vi "Message Check.vi"(8 "error in (no error)":errorcluster, 10 "element":cluster{"ID":string, "current time":timestamp}[](array[cluster]), 11 "Array in":refnum<class "Button.lvclass">[](array[class])) -> (0 "error out":errorcluster, 3 "Array":refnum<class "Button.lvclass">[](array[class]))   [LabVIEW 2018]
uses:
  Button Class/Button.lvclass
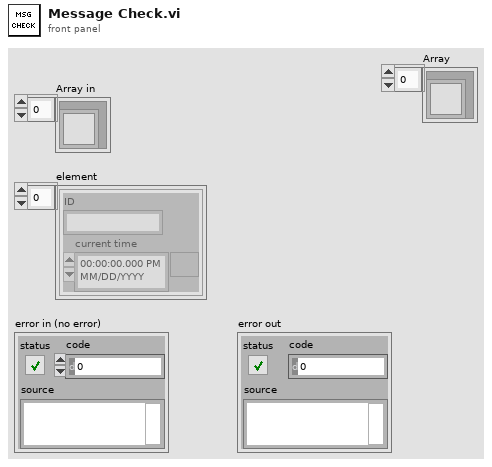
[diagram p1: front panel]
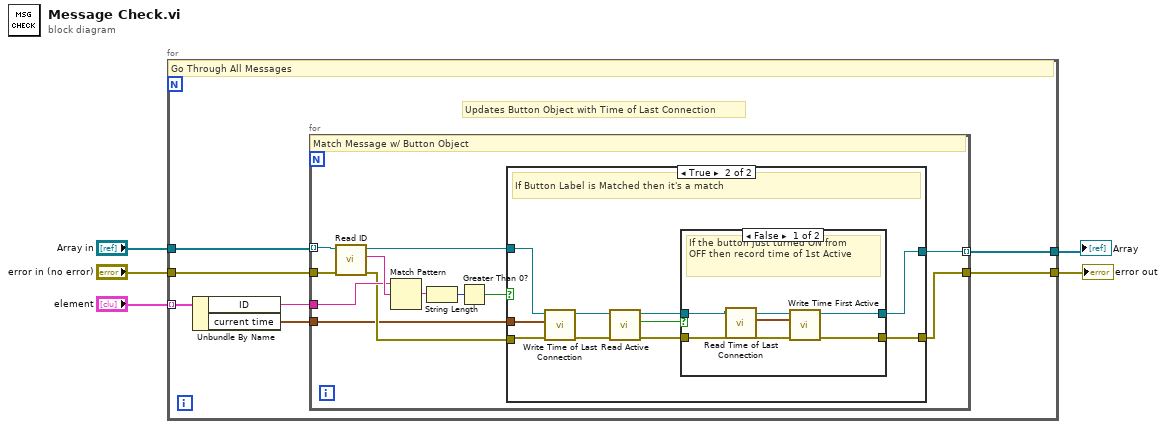
[diagram p0: block diagram]
diagram:
  n1 = for {
    tunnel: "element" -> [w12] mode=indexing
    tunnel: "Array in" -> [w11]
    tunnel: [w8] -> w5
    tunnel: "error in (no error)" -> [w7]
    tunnel: [w6] -> w1
    # "Updates Button Object with Time of Last Connection"
    # "Go Through All Messages"
    n2 = Unbundle By Name(w12) -> ("ID"=w10:string, "current time"=w9:timestamp)
    n3 = for {
      tunnel: w11 -> [w24] mode=indexing
      tunnel: w10 -> [w21]
      tunnel: w9 -> [w16]
      tunnel: [w15] -> w8
      tunnel: w7 -> [w23]
      tunnel: [w13] -> w6 mode=indexing
      # "Match Message w/ Button Object"
      n4 = call-dynamic "Read ID.vi"("error in (no error)"=w23, "Button in"=w24) -> ("error out"=w17:errorcluster, "ID"=w22:string, "Button out"=w18:refnum<class "Button.lvclass">)  [unwired: 7 in]
      n5 = Match Pattern(string=w21, regular expression=w22) -> (match substring=w19:string)  [unwired: 1 in, 3 out]
      n6 = String Length(string=w19) -> (length=w20:i32)
      n7 = Greater Than 0?(x=w20) -> (x > 0?=w14:bool)
      n8 = case shown="True" w14 {
        tunnel: w18 -> [w25 w36]
        tunnel: w17 -> [w26 w35]
        tunnel: w16 -> [_ w34]
        tunnel: [w26 w28] -> w15
        tunnel: [w25 w27] -> w13
        frame False {
          # "Not a Match"
        }
        frame True {
          # "If Button Label is Matched then it's a match"
          n9 = call-dynamic "Write Time of Last Connection.vi"("error in (no error)"=w35, "Time of Last Connection"=w34, "Button in"=w36) -> ("error out"=w33:errorcluster, "Button out"=w32:refnum<class "Button.lvclass">)  [unwired: 7 in]
          n10 = call-dynamic "Read Active.vi"("error in (no error)"=w33, "Button in"=w32) -> ("error out"=w29:errorcluster, "Active"=w31:bool, "Button out"=w30:refnum<class "Button.lvclass">)  [unwired: 7 in]
          n11 = case shown="False" w31 {
            tunnel: w30 -> [w42 w44]
            tunnel: w29 -> [w41 w45]
            tunnel: [w43 w45] -> w28
            tunnel: [w37 w44] -> w27
            frame False {
              # "If the button just turned ON from\nOFF then record time of 1st Active"
              n12 = call-dynamic "Read Time of Last Connection.vi"("error in (no error)"=w41, "Button in"=w42) -> ("error out"=w38:errorcluster, "Time of Last Connection"=w39:timestamp, "Button out"=w40:refnum<class "Button.lvclass">)  [unwired: 7 in]
              n13 = call-dynamic "Write Time First Active.vi"("error in (no error)"=w38, "Time First Active"=w39, "Button in"=w40) -> ("error out"=w43:errorcluster, "Button out"=w37:refnum<class "Button.lvclass">)  [unwired: 7 in]
            }
            frame True {
            }
          }
        }
      }
    }
  }
  "error out" <- w5
  "Array" <- w1
